vi "VG_PARK.vi"() -> ()   [LabVIEW 2020]
panel:
  out "PARK":bool
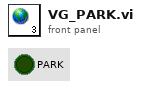
[diagram p1: front panel]
diagram:
